vi "Build Assert VI Path.vi"(6 "Assert VI path":path, 7 "Type":T1, 8 "error in (no error)":errorcluster, 10 "Template Path":path) -> (0 "error out":errorcluster)   [LabVIEW 2016]
doc: "Creates a new vi based on the specified template and saves it to the new path"
uses:
  <vilib>/Utility/Data Type/Type Definitions/Data Type.ctl
  <vilib>/Utility/Data Type/NI_Data Type.lvlib
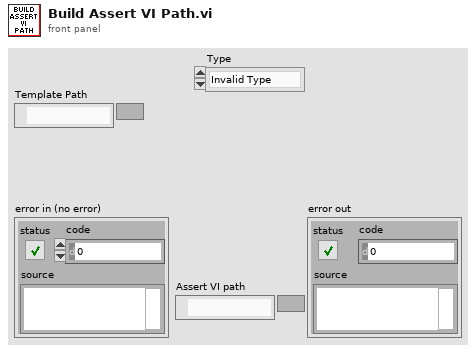
[diagram p1: front panel]
types:
  T1 = typedef "NI_Data Type.lvlib/Data Type.ctl" = enum8{"Invalid Type", "Void", "I8", "I16", "I32", "I64", "U8", "U16", "U32", "U64", "Single Float", "Double Float", "Extended Float", "Single Complex", "Double Complex", "Extended Complex", "Enum U8", "Enum U16", "Enum U32", "Enum U64", "Single Float With Unit", "Double Float With Unit", "Extended Float With Unit", "Single Complex with Unit", "Double Complex with Unit", "Extended Complex with Unit", "Boolean", "String", "Path", "Picture", "Tag", "Array", "Cluster", "Variant", "LV Variant", "Waveform", "Timestamp", "Digital Waveform", "Digital Data", "ExpressData", "Refnum", "External Data", "VI", "Poly VI", "LabVIEW Class Instance", "Fixed Point"}
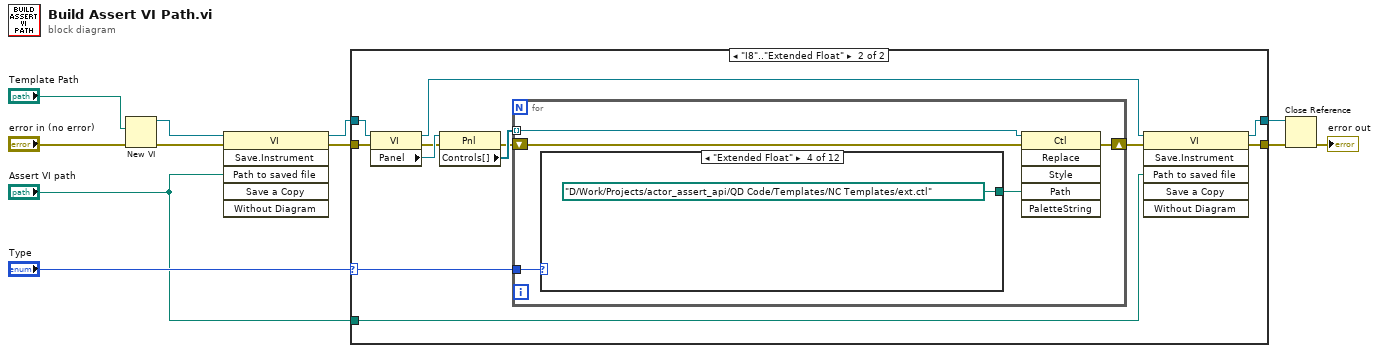
[diagram p0: block diagram]
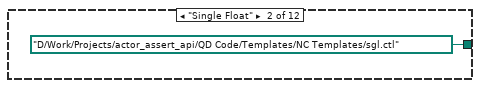
[diagram p4: hidden frame]
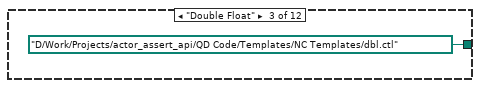
[diagram p5: hidden frame]
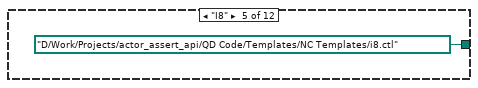
[diagram p6: hidden frame]
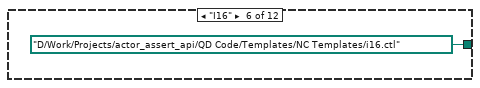
[diagram p7: hidden frame]
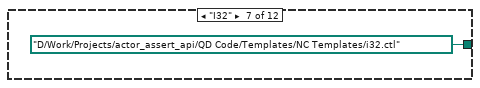
[diagram p8: hidden frame]
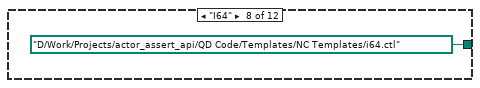
[diagram p9: hidden frame]
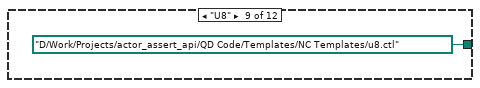
[diagram p10: hidden frame]
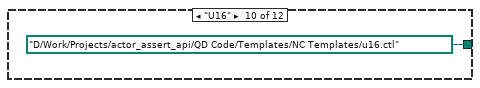
[diagram p11: hidden frame]
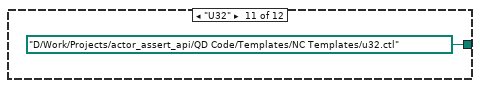
[diagram p12: hidden frame]
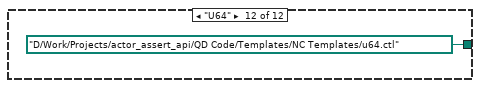
[diagram p13: hidden frame]
diagram:
  n1 = New VI(8:"error in (no error)", 10:"Template Path") -> (0:w8:errorcluster, 3:w7:refnum<vi>)  [unwired: 5 in]
  n2 = invoke class="VI" method="Save.Instrument"(reference=w7, error in=w8, "Path to saved file"="Assert VI path") -> (reference out=w4:refnum<vi>, error out=w2:errorcluster)  [unwired: 3 in, 4 out]
  n3 = case shown="\"I8\"..\"Extended Float\"" "Type" {
    selector: "Type" -> [_ w14]
    tunnel: [w13 w16] -> w5
    tunnel: w4 -> [w13 w25]
    tunnel: [w12 w18] -> w3
    tunnel: w2 -> [w12 w19]
    tunnel: "Assert VI path" -> [_ w15]
    frame Default {
    }
    frame "I8".."Extended Float" {
      n4 = property class="VI"(reference=w25, error in=w19) -> (reference out=w17:refnum<vi>, error out=w20:errorcluster, "Panel"=w24:refnum<vi>)
      n5 = property class="Pnl"(reference=w24, error in=w20) -> (error out=w21:errorcluster, "Controls[]"=w23:refnum<vi>[])  [unwired: 1 out]
      n6 = for {
        tunnel: w23 -> [w30] mode=indexing
        shift-right: [w28] -> w22
        shift-left: w21 -> [w27]
        tunnel: w14 -> [w26]
        n7 = case shown="\"Extended Float\"" w26 {
          tunnel: [_ path "D:/Work/Projects/actor_assert_api/QD Code/Templates/NC Templates/sgl.ctl" ("Path") path "D:/Work/Projects/actor_assert_api/QD Code/Templates/NC Templates/dbl.ctl" ("Path") path "D:/Work/Projects/actor_assert_api/QD Code/Templates/NC Templates/ext.ctl" ("Path") path "D:/Work/Projects/actor_assert_api/QD Code/Templates/NC Templates/i8.ctl" ("Path") path "D:/Work/Projects/actor_assert_api/QD Code/Templates/NC Templates/i16.ctl" ("Path") path "D:/Work/Projects/actor_assert_api/QD Code/Templates/NC Templates/i32.ctl" ("Path") path "D:/Work/Projects/actor_assert_api/QD Code/Templates/NC Templates/i64.ctl" ("Path") path "D:/Work/Projects/actor_assert_api/QD Code/Templates/NC Templates/u8.ctl" ("Path") path "D:/Work/Projects/actor_assert_api/QD Code/Templates/NC Templates/u16.ctl" ("Path") path "D:/Work/Projects/actor_assert_api/QD Code/Templates/NC Templates/u32.ctl" ("Path") path "D:/Work/Projects/actor_assert_api/QD Code/Templates/NC Templates/u64.ctl" ("Path")] -> w29
          frame Default {
          }
          frame "Single Float" {
          }
          frame "Double Float" {
          }
          frame "Extended Float" {
          }
          frame "I8" {
          }
          frame "I16" {
          }
          frame "I32" {
          }
          frame "I64" {
          }
          frame "U8" {
          }
          frame "U16" {
          }
          frame "U32" {
          }
          frame "U64" {
          }
        }
        n8 = invoke class="Ctl" method="Replace"(reference=w30, error in=w27, "Path"=w29) -> (error out=w28:errorcluster)  [unwired: 3 in, 5 out]
      }
      n9 = invoke class="VI" method="Save.Instrument"(reference=w17, error in=w22, "Path to saved file"=w15) -> (reference out=w16:refnum<vi>, error out=w18:errorcluster)  [unwired: 3 in, 4 out]
    }
  }
  n10 = Close Reference(reference=w5, error in (no error)=w3) -> (error out=→"error out":errorcluster)
